vi "Generic FXP Up Converter.vi"() -> ()   [LabVIEW 2010]
uses:
  FXP Type.ctl
panel:
  in  "Reset?":bool
  in  "Increment?":bool
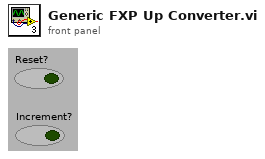
[diagram p1: front panel]
types:
  T1 = typedef "FXP Type.ctl" = fxp<+,6,6>
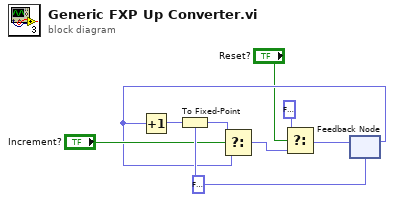
[diagram p0: block diagram]
diagram:
  w8 = T1 0.0 ("Counter FXP Type")
  n1 = feedback #1(w8) -> (w5:T1)
  n2 = Increment(x=w5) -> (x+1=w9:fxp<+,7,7>)
  n3 = To Fixed-Point(fixed-point type=w8, number=w9) -> (fixed-point=w7:T1)
  n4 = Select(t=w7, s="Increment?", f=w5) -> (s? t:f=w3:T1)
  n5 = Select(t=T1 0.0, s="Reset?", f=w3) -> (s? t:f=w1:T1)
  n6 = feedback-in #1(w1) -> ()
